vi "List Table.vi"(8 "error in (no error)":errorcluster, 11 "Access in":refnum<class "Access.lvclass">) -> (0 "error out":errorcluster, 2 "List Table":string[](array[string]), 3 "Access out":refnum<class "Access.lvclass">)   [LabVIEW 2021, in "Database.lvlib" / "Access.lvclass"]
uses:
  Access.lvclass
  Access.lvclass/Access.ctl
  <vilib>/addons/database/NI_Database_API.lvlib
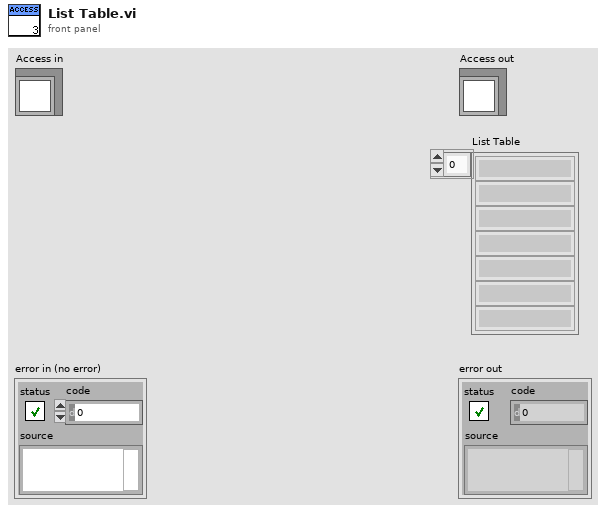
[diagram p1: front panel]
types:
  T1 = typedef "NI_Database_API.lvlib/Conn ObjectReference.ctl" = refnum<k1>
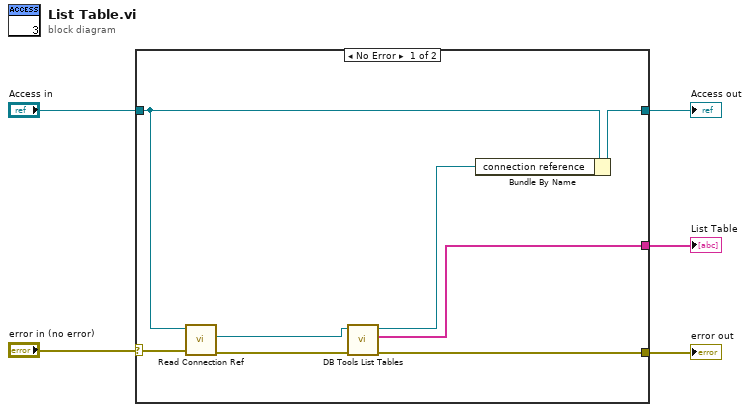
[diagram p0: block diagram]
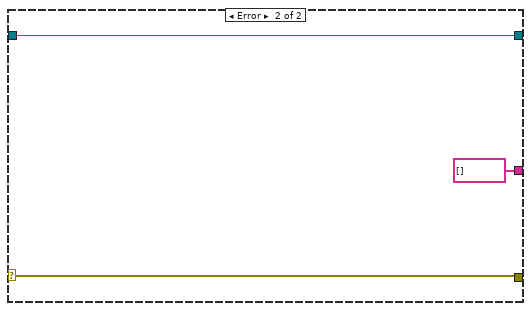
[diagram p2: hidden frame]
diagram:
  n1 = case shown="No Error" "error in (no error)" {
    selector: "error in (no error)" -> [w13 w15]
    tunnel: "Access in" -> [w10 w16]
    tunnel: [w8 w16] -> w3
    tunnel: [w9 w15] -> w2
    tunnel: [w6 string[] [] ("tables")] -> w1
    frame No Error {
      n2 = call-dynamic "Read Connection Ref.vi"("error in (no error)"=w13, "Access in"=w10) -> ("error out"=w12:errorcluster, "connection reference"=w11:T1)  [unwired: 7 in, 1 out]
      n3 = call <vilib>:"DB Tools List Tables.vi"("error in (no error)"=w12, "connection reference"=w11) -> ("error out"=w9:errorcluster, "tables"=w6:string[], "connection reference out"=w7:T1)  [unwired: 3 in]
      n4 = Bundle By Name(cluster=w10, "connection reference"=w7) -> (w8:refnum<class "Access.lvclass">)
    }
    frame Error {
    }
  }
  "error out" <- w2
  "Access out" <- w3
  "List Table" <- w1
